vi "Settings.vi"() -> ()   [LabVIEW 2013]
uses:
  qwtb_lvlib/TD GUI Settings.ctl
  qwtb_lvlib/TD Backend Engine.ctl
  qwtb_lvlib/TD Calculation Settings.ctl
  qwtb_lvlib/TD Uncertainty Calculation Method.ctl
  qwtb_lvlib/TD Correlation Calculation Settings.ctl
  qwtb_lvlib/TD DOF Calculation Settings.ctl
  qwtb_lvlib/TD MCM Calculation Settings.ctl
  qwtb_lvlib/TD MCM Calculation Method.ctl
  globals.vi
  <vilib>/Utility/xml.llb/Write to XML File(string).vi
  <vilib>/Utility/xml.llb/Read From XML File(string).vi
panel:
  out "Save data format":T9={"GUI Settings"={"Backend engine"=enum."Matlab by Script node", "QWTB Folder Path"=path ""}, "Calculation Settings"={"Verbose"=FALSE, "Uncertainty Calculation Method"=enum."none", "Correlations"={"Required"=FALSE, "Generate"=FALSE}, "Degrees of Freedom"={"Required"=FALSE, "Generate"=FALSE}, "MCM Calculation Settings"={"Repeats"=0, "Verbose"=FALSE, "Parallelization method"=enum."Single Core", "Processors"=0, "Temporary directory"="", "Randomize"=FALSE}}} {"Calculation Settings"."MCM Calculation Settings"."Processors" min=1 step=1; "Calculation Settings"."MCM Calculation Settings"."Repeats" min=1 step=1}
  in  "load":bool
  in  "save":bool
  in  "tmp dir":bool
  in  "close":bool
  in  "Calculation Settings":T3={"Verbose"=TRUE, "Uncertainty Calculation Method"=enum."none", "Correlations"={"Required"=FALSE, "Generate"=TRUE}, "Degrees of Freedom"={"Required"=TRUE, "Generate"=TRUE}, "MCM Calculation Settings"={"Repeats"=100, "Verbose"=TRUE, "Parallelization method"=enum."Single Core", "Processors"=1, "Temporary directory"=".", "Randomize"=TRUE}} {"MCM Calculation Settings"."Processors" min=1 step=1; "MCM Calculation Settings"."Repeats" min=1 step=1 format="%.0p"}
  in  "GUI Settings":T1={"Backend engine"=enum."Matlab by Script node", "QWTB Folder Path"=path ""}
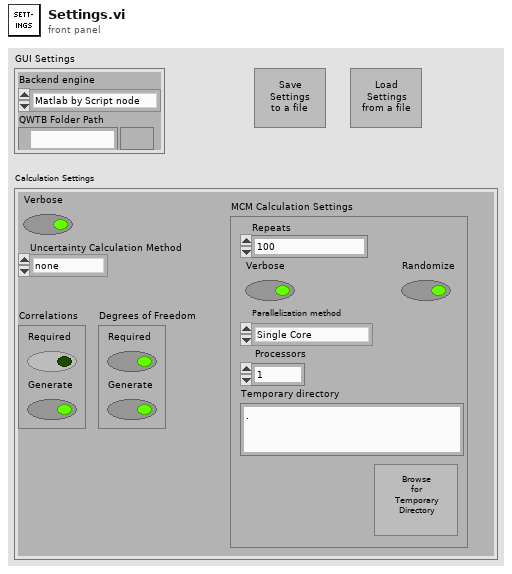
[diagram p1: front panel]
types:
  T1 = typedef "TD GUI Settings.ctl" = cluster{"Backend engine":T2, "QWTB Folder Path":path}
  T2 = typedef "TD Backend Engine.ctl" = enum16{"Matlab by Script node", "GNU Octave by GOLPI"}
  T3 = typedef "TD Calculation Settings.ctl" = cluster{"Verbose":bool, "Uncertainty Calculation Method":T4, "Correlations":T5, "Degrees of Freedom":T6, "MCM Calculation Settings":T7}
  T4 = typedef "TD Uncertainty Calculation Method.ctl" = enum16{"none", "GUF", "MCM"}
  T5 = typedef "TD Correlation Calculation Settings.ctl" = cluster{"Required":bool, "Generate":bool}
  T6 = typedef "TD DOF Calculation Settings.ctl" = cluster{"Required":bool, "Generate":bool}
  T7 = typedef "TD MCM Calculation Settings.ctl" = cluster{"Repeats":i32, "Verbose":bool, "Parallelization method":T8, "Processors":i32, "Temporary directory":string, "Randomize":bool}
  T8 = typedef "TD MCM Calculation Method.ctl" = enum16{"Single Core", "Multi Core", "Multi Station"}
  T9 = cluster{"GUI Settings":T1, "Calculation Settings":T3}
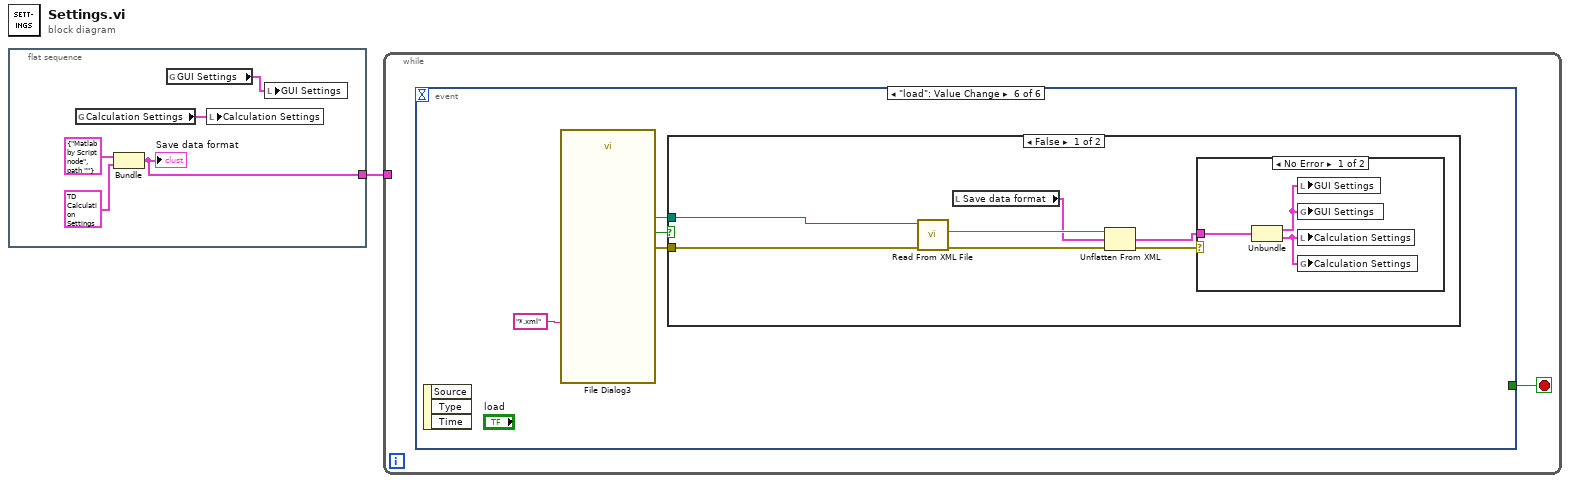
[diagram p0: block diagram]
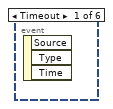
[diagram p2: hidden frame]
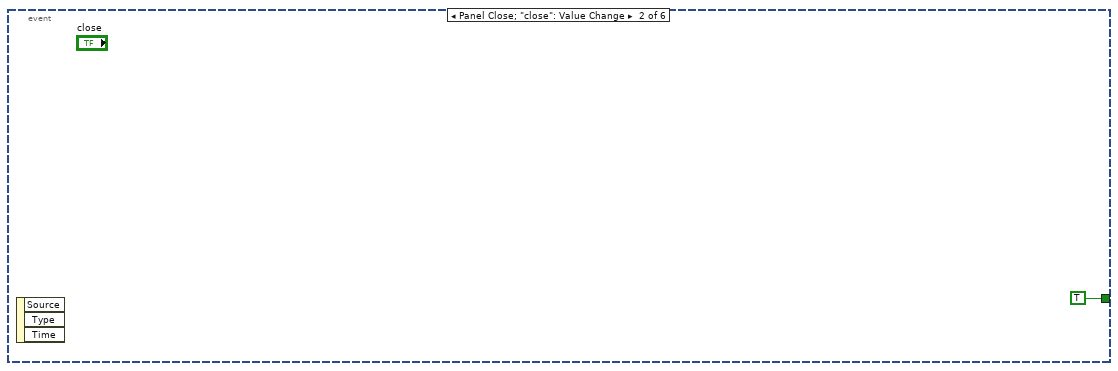
[diagram p3: hidden frame]
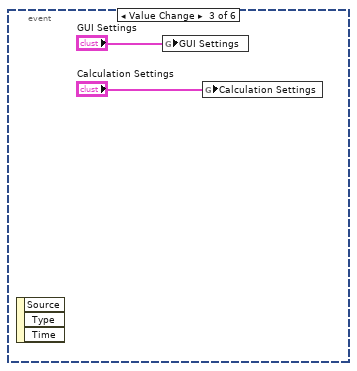
[diagram p4: hidden frame]
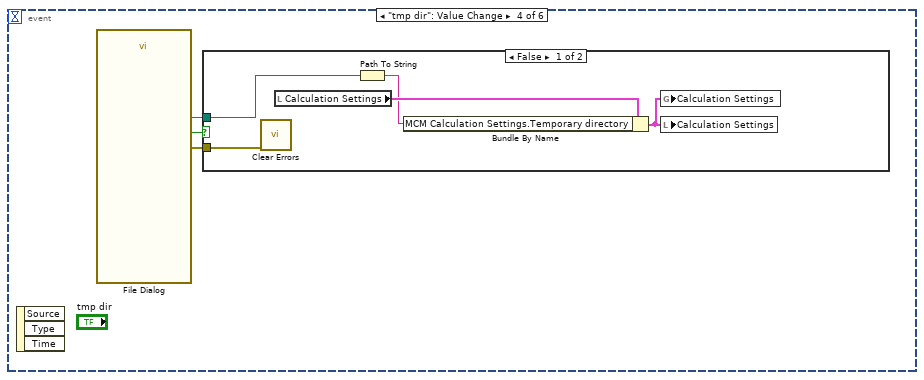
[diagram p5: hidden frame]
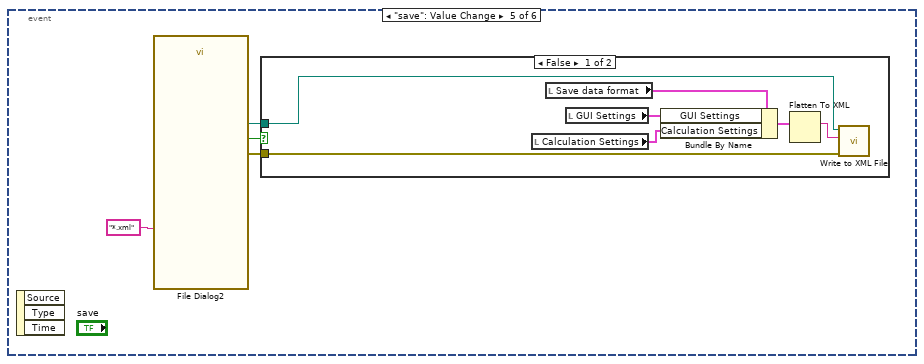
[diagram p7: hidden frame]
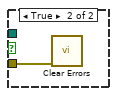
[diagram p8: hidden frame]
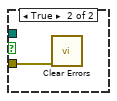
[diagram p10: hidden frame]
diagram:
  n1 = flat-sequence {
    tunnel: [w2] -> w1
    frame #0 {
      n2 = global read "globals.vi" "Calculation Settings"() -> (w6:T3)
      n3 = Bundle("GUI Settings"=T1 {"Backend engine"=enum."Matlab by Script node", "QWTB Folder Path"=path ""}, "Calculation Settings"=T3 {"Verbose"=TRUE, "Uncertainty Calculation Method"=enum."none", "Correlations"={"Required"=FALSE, "Generate"=TRUE}, "Degrees of Freedom"={"Required"=TRUE, "Generate"=TRUE}, "MCM Calculation Settings"={"Repeats"=100, "Verbose"=TRUE, "Parallelization method"=enum."Single Core", "Processors"=1, "Temporary directory"=".", "Randomize"=TRUE}}) -> (w2:T9)  [unwired: 1 in]
      "Save data format" <- w2
      n4 = global read "globals.vi" "GUI Settings"() -> (w5:T1)
      n5 = local write "Calculation Settings"(w6) -> ()
      n6 = local write "GUI Settings"(w5) -> ()
    }
  }
  n7 = while {
    tunnel: w1 -> [_]
    stop <- w7 stop-if-true
    n8 = event shown="[5] \"load\": Value Change" {
      selector: _ -> [_ _ _ _ _ _]
      dyn-events: _ -> [_ _ _ _ _ _]
      timeout: _ -> [_ _ _ _ _ _]
      tunnel: [_ TRUE ("cancel") _ _ _ _] -> w7
      event Timeout {
        n9 = event-data() -> ()  [unwired: 1 in, 3 out]
      }
      event Panel Close; "close": Value Change {
        n10 = event-data() -> ()  [unwired: 1 in, 3 out]
      }
      event Value Change {
        n11 = event-data() -> ()  [unwired: 1 in, 3 out]
        n12 = global write "globals.vi" "GUI Settings"("GUI Settings") -> ()
        n13 = global write "globals.vi" "Calculation Settings"("Calculation Settings") -> ()
      }
      event "tmp dir": Value Change {
        n14 = event-data() -> ()  [unwired: 1 in, 3 out]
        n15 = call "File Dialog"() -> ("selected path"=w13:path, "cancelled"=w12:bool, "error out"=w11:errorcluster)  [unwired: 12 in, 1 out]
        n16 = case shown="False" w12 {
          tunnel: w13 -> [w18 _]
          tunnel: w11 -> [w14 _]
          frame False {
            n17 = call <vilib>:"Clear Errors.vi"("error in (no error)"=w14) -> ()  [unwired: 6 in, 1 out]
            n18 = local read "Calculation Settings"() -> (w17:T3)
            n19 = Path To String(path=w18) -> (string=w16:string)
            n20 = Bundle By Name(cluster=w17, "MCM Calculation Settings.Temporary directory"=w16) -> (w15:T3)
            n21 = global write "globals.vi" "Calculation Settings"(w15) -> ()
            n22 = local write "Calculation Settings"(w15) -> ()
          }
          frame True {
          }
        }
      }
      event "save": Value Change {
        n23 = event-data() -> ()  [unwired: 1 in, 3 out]
        n24 = call "File Dialog2"("pattern (all files)"="*.xml") -> ("selected path"=w19:path, "cancelled"=w21:bool, "error out"=w20:errorcluster)  [unwired: 11 in, 1 out]
        n25 = case shown="False" w21 {
          tunnel: w20 -> [w28 w30]
          tunnel: w19 -> [w29 _]
          frame False {
            n26 = local read "Calculation Settings"() -> (w25:T3)
            n27 = local read "Save data format"() -> (w23:T9)
            n28 = local read "GUI Settings"() -> (w26:T1)
            n29 = Bundle By Name(cluster=w23, "GUI Settings"=w26, "Calculation Settings"=w25) -> (w24:T9)
            n30 = Flatten To XML(anything=w24) -> (xml string=w27:string)
            n31 = call-poly <vilib>:"Write to XML File.vi"("error in (no error)"=w28, "XML Input"=w27, "XML File Path"=w29) -> ()  [unwired: 6 in, 3 out]
          }
          frame True {
            n32 = call <vilib>:"Clear Errors.vi"("error in (no error)"=w30) -> ()  [unwired: 6 in, 1 out]
          }
        }
      }
      event "load": Value Change {
        n33 = event-data() -> ()  [unwired: 1 in, 3 out]
        n34 = call "File Dialog3"("pattern (all files)"="*.xml") -> ("selected path"=w31:path, "cancelled"=w33:bool, "error out"=w32:errorcluster)  [unwired: 11 in, 1 out]
        n35 = case shown="False" w33 {
          tunnel: w32 -> [w40 w45]
          tunnel: w31 -> [w41 _]
          frame False {
            n36 = call-poly <vilib>:"Read From XML File.vi"("error in (no error)"=w40, "XML File Path"=w41) -> ("error out"=w38:errorcluster, "XML Elements"=w39:string)  [unwired: 7 in, 1 out]
            n37 = local read "Save data format"() -> (w35:T9)
            n38 = Unflatten From XML(xml string=w39, type=w35, error in (no error)=w38) -> (value=w36:T9, error out=w37:errorcluster)
            n39 = case shown="No Error" w37 {
              tunnel: w36 -> [w44 _]
              frame No Error {
                n40 = Unbundle(w44) -> ("GUI Settings"=w43:T1, "Calculation Settings"=w42:T3)
                n41 = local write "GUI Settings"(w43) -> ()
                n42 = global write "globals.vi" "GUI Settings"(w43) -> ()
                n43 = local write "Calculation Settings"(w42) -> ()
                n44 = global write "globals.vi" "Calculation Settings"(w42) -> ()
              }
              frame Error {
              }
            }
          }
          frame True {
            n45 = call <vilib>:"Clear Errors.vi"("error in (no error)"=w45) -> ()  [unwired: 6 in, 1 out]
          }
        }
      }
    }
  }
